vi "parse.series.vi"(8 "error in":errorcluster, 11 "string in":string) -> (0 "error out":errorcluster, 3 "series json":T1)   [LabVIEW 2024]
uses:
  <vilib>/addons/_JKI.lib/Serialization/JSON/JKI JSON Serialization.lvlib
  TypeDefs/series--cluster.ctl
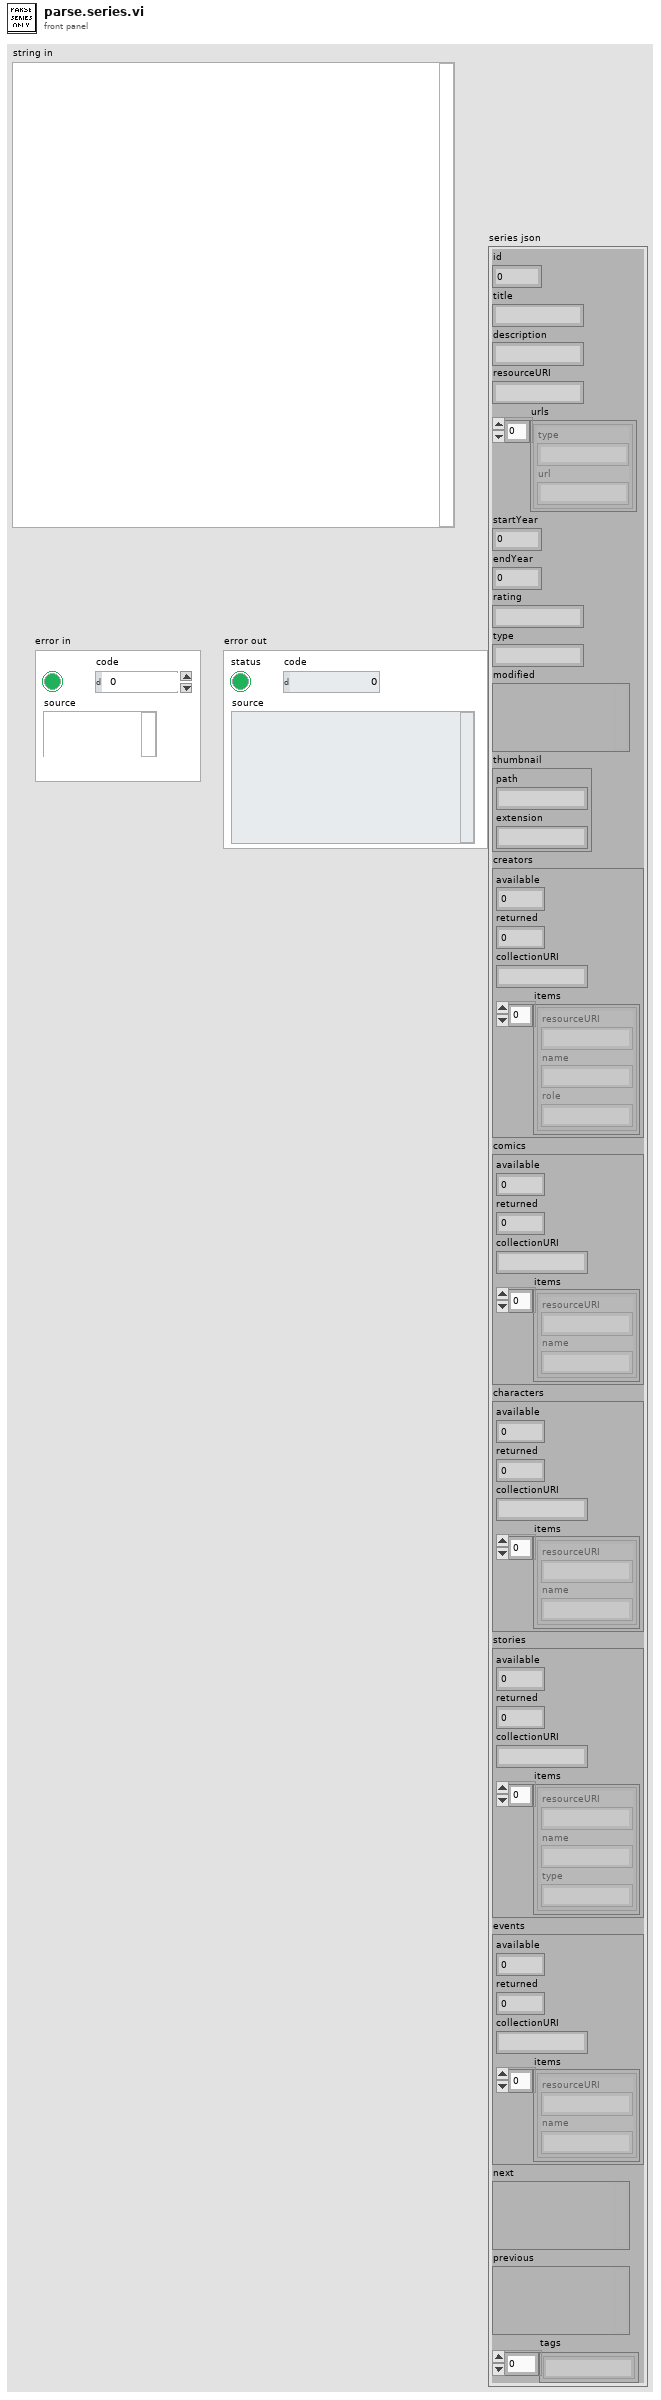
[diagram p1: front panel]
types:
  T1 = typedef "series--cluster.ctl" = cluster{"id":i32, "title":string, "description":string, "resourceURI":string, "urls":cluster{"type":string, "url":string}[], "startYear":i32, "endYear":i32, "rating":string, "type":string, "modified":variant, "thumbnail":cluster{"path":string, "extension":string}, "creators":cluster{"available":i32, "returned":i32, "collectionURI":string, "items":cluster{"resourceURI":string, "name":string, "role":string}[]}, "comics":cluster{"available":i32, "returned":i32, "collectionURI":string, "items":cluster{"resourceURI":string, "name":string}[]}, "characters":cluster{"available":i32, "returned":i32, "collectionURI":string, "items":cluster{"resourceURI":string, "name":string}[]}, "stories":cluster{"available":i32, "returned":i32, "collectionURI":string, "items":cluster{"resourceURI":string, "name":string, "type":string}[]}, "events":cluster{"available":i32, "returned":i32, "collectionURI":string, "items":cluster{"resourceURI":string, "name":string}[]}, "next":variant, "previous":variant, "tags":string[]}
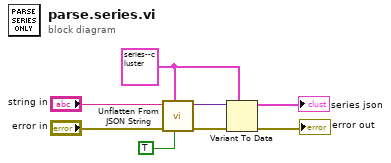
[diagram p0: block diagram]
diagram:
  w2 = T1 {"id"=0, "title"="", "description"="", "resourceURI"="", "urls"=[], "startYear"=0, "endYear"=0, "rating"="", "type"="", "modified"=variant, "thumbnail"={"path"="", "extension"=""}, "creators"={"available"=0, "returned"=0, "collectionURI"="", "items"=[]}, "comics"={"available"=0, "returned"=0, "collectionURI"="", "items"=[]}, "characters"={"available"=0, "returned"=0, "collectionURI"="", "items"=[]}, "stories"={"available"=0, "returned"=0, "collectionURI"="", "items"=[]}, "events"={"available"=0, "returned"=0, "collectionURI"="", "items"=[]}, "next"=variant, "previous"=variant, "tags"=[]} ("Cluster")
  n1 = call <vilib>:"Unflatten From JSON String.vi"("Nulls as Defaults (F)"=TRUE, "Type and Defaults"=w2, "error in (no error)"="error in", "JSON String"="string in") -> ("error out"=w5:errorcluster, "Variant"=w6:variant)  [unwired: 6 in]
  n2 = Variant To Data(error in=w5, type=w2, Variant=w6) -> (data=→"series json":T1, error out=→"error out":errorcluster)
